vi "Localization.vi"() -> ()   [LabVIEW 2023, in "Caller B.lvlib" / "Caller B.lvclass"]
uses:
  Caller B/Caller B/Caller B.lvclass
panel:
  in  "value retrieved":string="Value retrieved: %f\n"
  in  "begin":string="Begin log.\n"
  in  "request golden ratio":string="Request value of golden ratio.\n"
  in  "request e":string="Request value of e.\n"
  in  "request pi":string="Request value of pi.\n"
  in  "actor stopped":string="Actor stopped.\n"
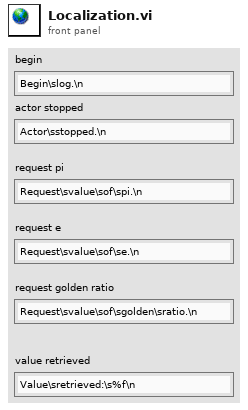
[diagram p1: front panel]
diagram:
